vi "ValueChange.vi"(11 "Int":ext) -> (3 "Changed":bool)   [LabVIEW 2019]
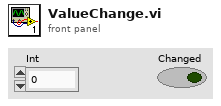
[diagram p1: front panel]
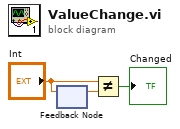
[diagram p0: block diagram]
diagram:
  n1 = feedback #1() -> (w1:ext)  [unwired: 1 in]
  n2 = feedback-in #1("Int") -> ()
  n3 = Not Equal?(x="Int", y=w1) -> (x != y?=→"Changed":bool)
